vi "New Listbox Item Names Binding.vi"(9 "Set To Top?":T1, 10 "LstBox Refnum":refnum<vi>) -> (0 "error out":errorcluster, 3 "MCListboxItemNamesBinding":refnum<class "ListboxItemNamesBinding.lvclass">)   [LabVIEW 2017, in "Transport.lvlib" / "ListboxItemNamesBinding.lvclass"]
doc: "<License>\nCopyright © 2017 Composed Systems, LLC | All rights reserved\nwww.composed.io\n\nAuthor: Ethan Stern <ethan.stern@composed.io>\n\nThis software is provided \"AS IS\" WITHOUT WARRANTIES, either express or implied, AND IS FOR EDUCATIONAL PURPOSES ONLY.\n</License>"
uses:
  ListboxItemNamesBinding.lvclass
  MCListbox Binding Options.ctl
  ListboxItemNamesBinding.lvclass/ListboxItemNamesBinding.ctl
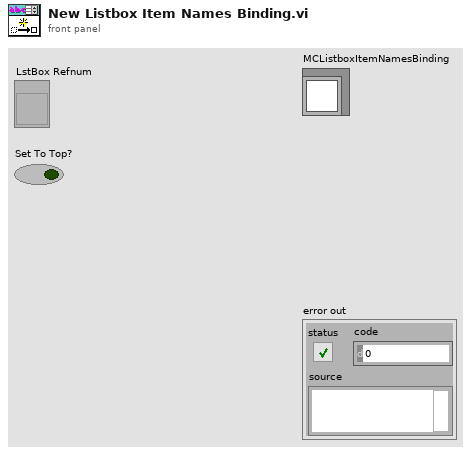
[diagram p1: front panel]
types:
  T1 = typedef "Transport.lvlib/ListboxItemNamesBinding.lvclass/MCListbox Binding Options.ctl" = bool
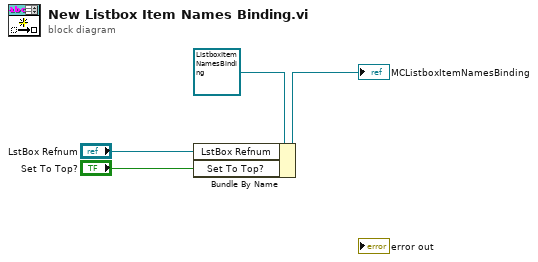
[diagram p0: block diagram]
diagram:
  n1 = Bundle By Name(cluster=refnum<class "ListboxItemNamesBinding.lvclass"> refnum ("TerminalBinding in"), "LstBox Refnum"="LstBox Refnum", "Set To Top?"="Set To Top?") -> (→"MCListboxItemNamesBinding":refnum<class "ListboxItemNamesBinding.lvclass">)
